vi "Call-CryptoNight-Step-3-Fpga.vi"(8 "error in":errorcluster, 9 "Data in":u8[](array[numeric]) format="%.0x", 10 "Size-in":i32, 11 "Command":u32[](array[numeric]) format="%.0x") -> (0 "error out":errorcluster, 1 "b_out":u64[](array[numeric]) format="%.0x", 2 "a_out":u64[](array[numeric]) format="%.0x", 3 "Data out":u8[](array[numeric]))   [LabVIEW 2017]
uses:
  <vilib>/rvi/interface/nirviOpenFPGA/nirviOpenFPGA.xnode
  FPGA/Fpga-Top-Level.vi
  <vilib>/rvi/interface/nirviMethod/nirviMethod.xnode
  <vilib>/rvi/interface/nirviReadWriteControl/nirviReadWriteControl.xnode
  NiFpgaLv.dll
  <vilib>/Utility/error.llb/Error Cluster From Error Code.vi
  <vilib>/rvi/interface/Simulation/niFpgaSimulationCallBeginRW.vi
  <vilib>/rvi/errors/niLvFpgaAdjustHostInterfaceError.vi
  <vilib>/FPGAPlugInAG/Dynamic/niLvFpga_WriteFifo_Dynamic.vi
  <vilib>/rvi/errors/niLvFpgaMergeErrorWithErrorCode.vi
  <vilib>/FPGAPlugInAG/Dynamic/niLvFpga_ReadFifo_Dynamic.vi
  <vilib>/rvi/interface/nirviCloseFPGA/nirviCloseFPGA.xnode
  <vilib>/FPGAPlugInAG/Dynamic/niLvFpga_Close_Dynamic.vi
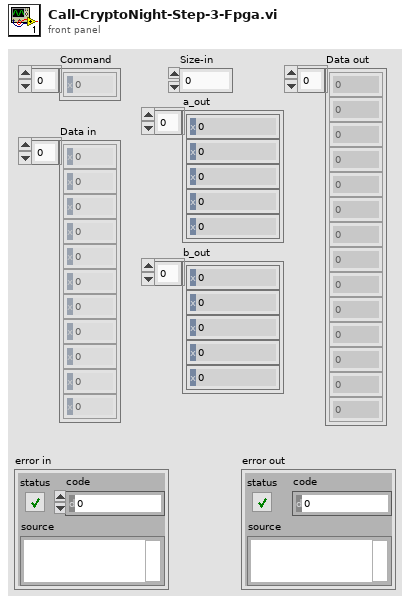
[diagram p1: front panel]
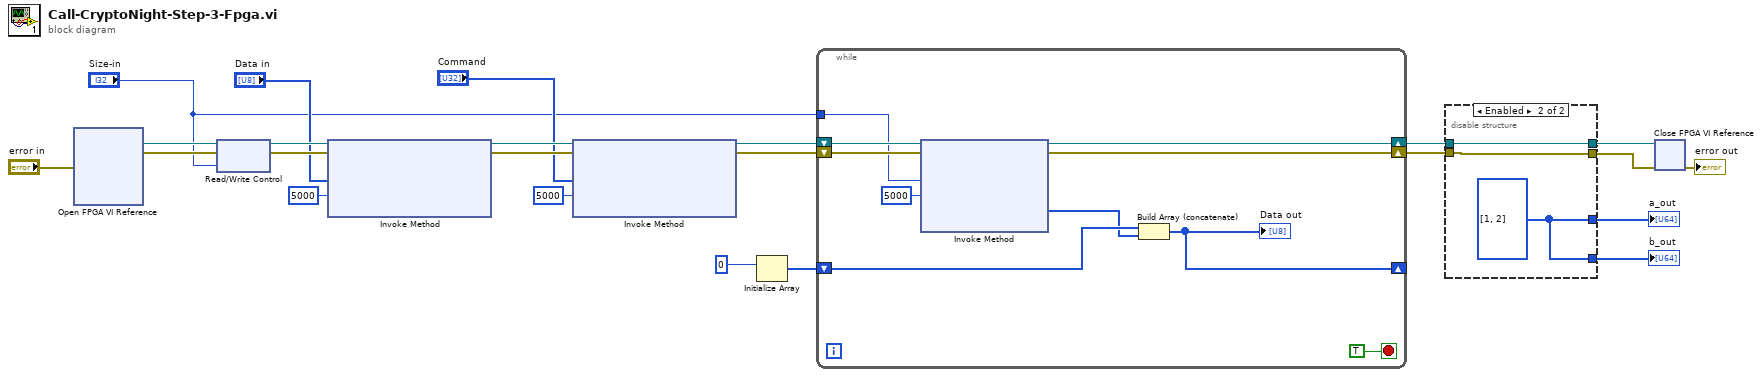
[diagram p0: block diagram]
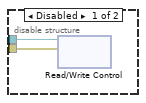
[diagram p2: hidden frame]
diagram:
  n1 = xnode "Open FPGA VI Reference"("error in"="error in") -> ("FPGA VI Reference Out"=w21:refnum<k20>, "error out"=w22:errorcluster)  [unwired: 1 in]
  n2 = xnode "Read/Write Control"("FPGA VI Reference In"=w21, "error in"=w22, "Size-in"="Size-in") -> ("FPGA VI Reference Out"=w20:refnum<k20>, "error out"=w19:errorcluster)
  n3 = xnode "Invoke Method"("FPGA VI Reference In"=w20, "error in"=w19, "Data"="Data in", "Timeout (ms)"=5000) -> ("FPGA VI Reference Out"=w16:refnum<k20>, "error out"=w15:errorcluster)  [unwired: 1 out]
  n4 = xnode "Invoke Method"("FPGA VI Reference In"=w16, "error in"=w15, "Data"="Command", "Timeout (ms)"=5000) -> ("FPGA VI Reference Out"=w12:refnum<k20>, "error out"=w11:errorcluster)  [unwired: 1 out]
  n5 = Initialize Array(u8 0) -> (w8:u8[])  [unwired: 1 in]
  n6 = while {
    shift-right: [w27] -> w5
    shift-left: w12 -> [w33]
    shift-right: [w26] -> w6
    shift-left: w11 -> [w32]
    tunnel: "Size-in" -> [w30]
    shift-right: [w25] -> _
    shift-left: w8 -> [w29]
    stop <- TRUE stop-if-true
    n7 = xnode "Invoke Method"("FPGA VI Reference In"=w33, "error in"=w32, "Number of Elements"=w30, "Timeout (ms)"=5000) -> ("FPGA VI Reference Out"=w27:refnum<k20>, "error out"=w26:errorcluster, "Data"=w28:u8[])  [unwired: 1 out]
    n8 = Build Array (concatenate)(w29, w28) -> (w25:u8[])
    "Data out" <- w25
  }
  n9 = disable-structure shown="Enabled" {
    disable-tunnel: w6 -> [w35 w37]
    disable-tunnel: w5 -> [w34 w38]
    disable-tunnel: [_ w38] -> w4
    disable-tunnel: [_ w37] -> w3
    disable-tunnel: [_ w36] -> w2
    disable-tunnel: [_ w36] -> w1
    frame Disabled {
      n10 = xnode "Read/Write Control"("FPGA VI Reference In"=w34, "error in"=w35) -> ()  [unwired: 1 in, 2 out]
    }
    frame Enabled {
      w36 = u64[] [1, 2] ("a_out")
    }
  }
  "a_out" <- w2
  "b_out" <- w1
  n11 = xnode "Close FPGA VI Reference"("FPGA VI Reference In"=w4, "error in"=w3) -> ("error out"=→"error out":errorcluster)
